vi "SV Limit Testing for Monitoring (N Ch) (waveform).vi"(7 "reset":bool, 9 "lower limit":dbl=-inf format="%.2f", 10 "upper limit":dbl=inf format="%.2f", 11 "input signals":waveform(dbl)[](array[waveform])) -> (1 "lower limit clearances":dbl[](array[numeric]) format="%.6f", 2 "upper limit clearances":dbl[](array[numeric]) format="%.6f", 3 "tests passed":bool[](array[boolean]), 5 "timestamps":timestamp[](array[timestamp]) format="%<%.6X\n%x>T")   [LabVIEW 2017]
doc: "Performs limit testing on waveforms, spectra, XY data, identified peaks, or scalar measurements. You can wire <B>output values</B> to a graph to view the limits, signal, and failures. Wire data to the<B> signal in</B> input to determine the polymorphic instance to use or manually select the instance."
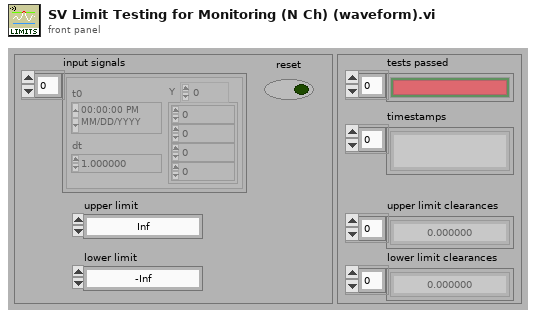
[diagram p1: front panel]
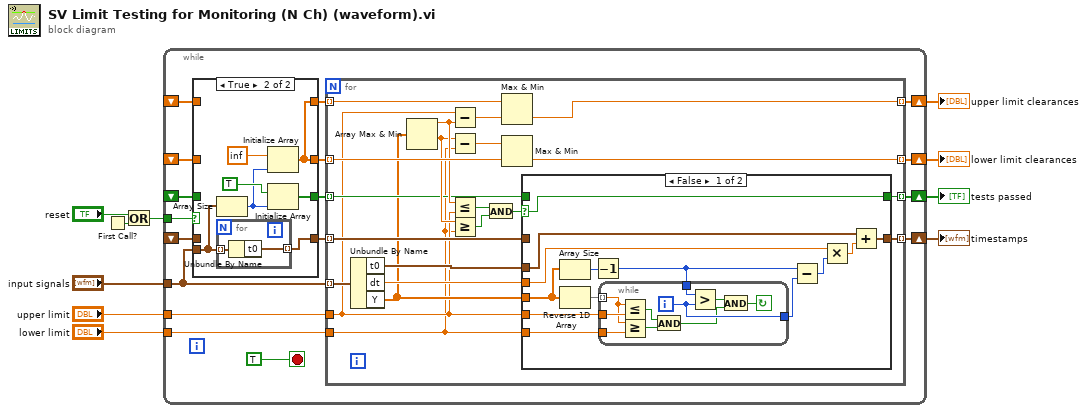
[diagram p0: block diagram]
diagram:
  n1 = First Call?() -> (First Call?: T/F=w3:bool)
  n2 = Or(x="reset", y=w3) -> (x .or. y?=w4:bool)
  n3 = while {
    tunnel: "input signals" -> [w13]
    tunnel: "upper limit" -> [w25]
    tunnel: "lower limit" -> [w22]
    shift-right: [w27] -> w8
    shift-left: _ -> [w20]
    shift-right: [w26] -> w7
    shift-left: _ -> [w19]
    shift-right: [w21] -> w6
    shift-left: _ -> [w18]
    shift-right: [w24] -> w2
    shift-left: _ -> [w12]
    tunnel: w4 -> [w17]
    stop <- TRUE stop-if-true
    n4 = case shown="True" w17 {
      tunnel: w20 -> [w31 _]
      tunnel: [w31 w32] -> w16
      tunnel: w19 -> [w30 _]
      tunnel: [w30 w32] -> w15
      tunnel: w18 -> [w29 _]
      tunnel: [w29 w36] -> w14
      tunnel: [w28 w38] -> w11
      tunnel: w13 -> [_ w37]
      tunnel: w12 -> [w28 _]
      frame False {
      }
      frame True {
        n5 = Array Size(array=w37) -> (size(s)=w33:i32)
        n6 = for {
          tunnel: w37 -> [w40] mode=indexing
          tunnel: [w39] -> w38 mode=indexing
          n7 = Unbundle By Name(w40) -> ("t0"=w39:timestamp)
        }
        n8 = Initialize Array(inf, w33) -> (w32:dbl[])
        n9 = Initialize Array(TRUE, w33) -> (w36:bool[])
      }
    }
    n10 = for {
      tunnel: w13 -> [w61] mode=indexing
      tunnel: [w60] -> w27 mode=indexing
      tunnel: [w59] -> w26 mode=indexing
      tunnel: w16 -> [w54] mode=indexing
      tunnel: w15 -> [w53] mode=indexing
      tunnel: w14 -> [w50] mode=indexing
      tunnel: w11 -> [w48] mode=indexing
      tunnel: w25 -> [w44]
      tunnel: [w41] -> w24 mode=indexing
      tunnel: w22 -> [w43]
      tunnel: [w42] -> w21 mode=indexing
      n11 = Unbundle By Name(w61) -> ("t0"=w47:timestamp, "dt"=w46:dbl, "Y"=w45:dbl[])
      n12 = Array Max & Min(array=w45) -> (max value=w52:dbl, min value=w51:dbl)  [unwired: 2 out]
      n13 = Subtract(x=w44, y=w52) -> (x-y=w56:dbl)
      n14 = Subtract(x=w51, y=w43) -> (x-y=w55:dbl)
      n15 = Less Or Equal?(x=w52, y=w44) -> (x <= y?=w58:bool)
      n16 = Greater Or Equal?(x=w51, y=w43) -> (x >= y?=w57:bool)
      n17 = And(x=w58, y=w57) -> (x .and. y?=w49:bool)
      n18 = Max & Min(x=w54, y=w56) -> (min(x,y)=w60:dbl)  [unwired: 1 out]
      n19 = Max & Min(x=w55, y=w53) -> (min(x,y)=w59:dbl)  [unwired: 1 out]
      n20 = case shown="False" w49 {
        selector: w49 -> [w71 _]
        tunnel: w48 -> [_ w86]
        tunnel: [w73 w86] -> w41
        tunnel: w47 -> [w74 _]
        tunnel: w46 -> [w70 _]
        tunnel: w50 -> [_ w85]
        tunnel: [w71 w85] -> w42
        tunnel: w45 -> [w62 _]
        tunnel: w44 -> [w69 _]
        tunnel: w43 -> [w68 _]
        frame False {
          n21 = Array Size(array=w62) -> (size(s)=w66:i32)
          n22 = Reverse 1D Array(array=w62) -> (reversed array=w67:dbl[])
          n23 = Decrement(x=w66) -> (x-1=w65:i32)
          n24 = while {
            tunnel: [w78] -> w64
            tunnel: w69 -> [w82]
            tunnel: w68 -> [w81]
            tunnel: w67 -> [w80] mode=indexing
            tunnel: w65 -> [w79]
            i -> [w78]
            stop <- w75 continue-if-true
            n25 = Less Or Equal?(x=w80, y=w82) -> (x <= y?=w84:bool)
            n26 = Greater Or Equal?(x=w80, y=w81) -> (x >= y?=w83:bool)
            n27 = And(x=w84, y=w83) -> (x .and. y?=w76:bool)
            n28 = Greater?(x=w79, y=w78) -> (0:w77:bool)
            n29 = And(x=w77, y=w76) -> (x .and. y?=w75:bool)
          }
          n30 = Subtract(x=w65, y=w64) -> (x-y=w63:i32)
          n31 = Multiply(x=w70, y=w63) -> (x*y=w72:dbl)
          n32 = Add(x=w74, y=w72) -> (x+y=w73:timestamp)
        }
        frame True {
        }
      }
    }
  }
  "tests passed" <- w6
  "upper limit clearances" <- w8
  "lower limit clearances" <- w7
  "timestamps" <- w2
